vi "PrependDUTID.vi"(10 "ECU Pin":string, 11 "Socket":u64) -> (3 "String":string)   [LabVIEW 2024, in "Shared Steps.lvlib"]
uses:
  Shared Steps.lvlib
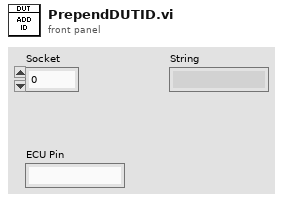
[diagram p1: front panel]
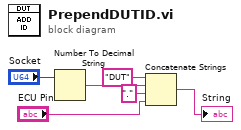
[diagram p0: block diagram]
diagram:
  n1 = Number To Decimal String(number="Socket") -> (decimal integer string=w2:string)  [unwired: 1 in]
  n2 = Concatenate Strings("DUT" ("string"), w2, "." ("string"), "ECU Pin") -> (→"String":string)
